vi "Test - LabVIEW-ini Config.vi"() -> ()   [LabVIEW 2021]
uses:
  Sources/Global Config.ctl
  Sources/ini Entry.ctl
  Sources/VIPM.ctl
panel:
  out "text":string
  out "Test Result":bool
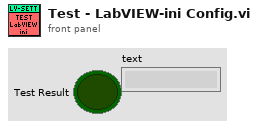
[diagram p1: front panel]
types:
  T1 = enum16{"open", "replace", "create", "open or create", "replace or create", "replace or create with confirmation"}
  T2 = typedef "ini Entry.ctl" = cluster{"section":string, "key":string, "value":variant}
  T3 = typedef "Global Config.ctl" = cluster{"LabVIEW.ini":T2[], "VIPM":T4}
  T4 = typedef "VIPM.ctl" = cluster{"official-packages":string[], "unofficial-package-urls":string[]}
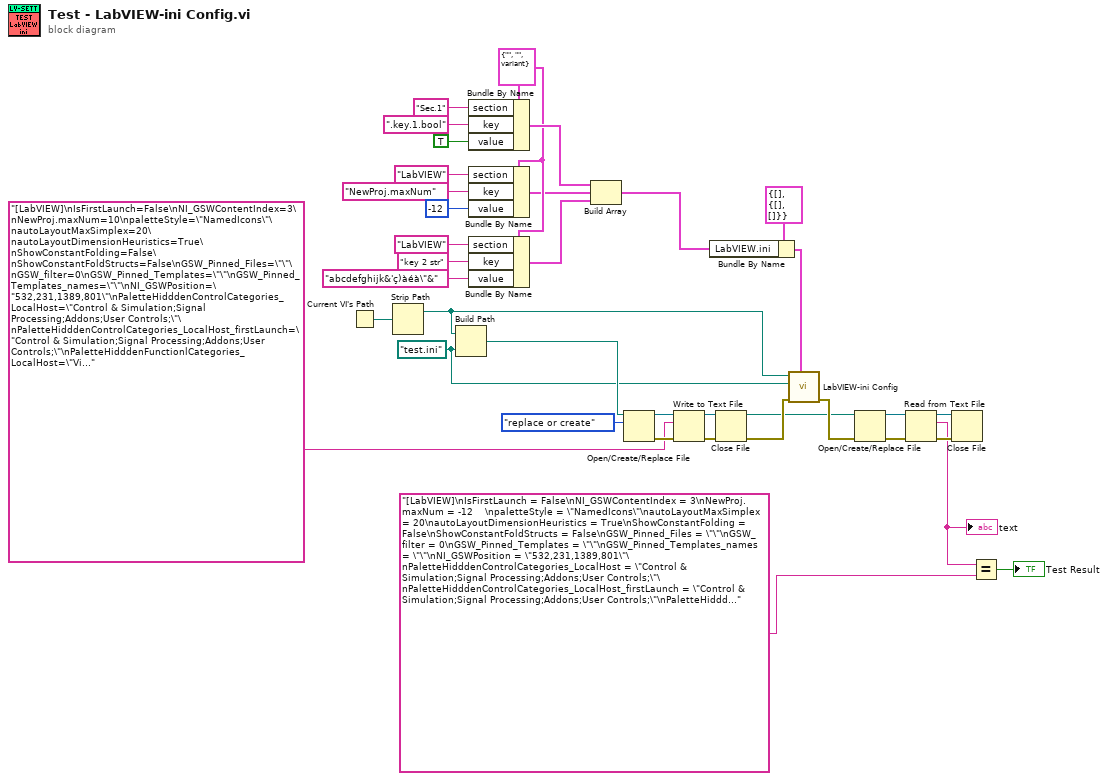
[diagram p0: block diagram]
diagram:
  w12 = path "test.ini" ("name or relative path")
  w24 = T2 {"section"="", "key"="", "value"=variant} ("ini Entry")
  n1 = Current VI's Path() -> (path=w20:path)
  n2 = Strip Path(path=w20) -> (stripped path=w14:path)  [unwired: 1 out]
  n3 = Build Path(base path=w14, name or relative path=w12) -> (appended path=w13:path)
  n4 = Bundle By Name(cluster=w24, "section"="Sec.1", "key"=".key.1.bool", "value"=TRUE) -> (w31:T2)
  n5 = Bundle By Name(cluster=w24, "section"="LabVIEW", "key"="NewProj.maxNum", "value"=-12) -> (w22:T2)
  n6 = Bundle By Name(cluster=w24, "section"="LabVIEW", "key"="key 2 str", "value"="abcdefghijk&'ç)àéà\"&" ("key")) -> (w21:T2)
  n7 = Build Array(w31, w22, w21) -> (w30:T2[])
  n8 = Open/Create/Replace File(file path (use dialog)=w13, operation (0:open)=T1."replace or create") -> (refnum out=w19:refnum<file>, error out=w18:errorcluster)  [unwired: 4 in, 1 out]
  n9 = Write to Text File(file (use dialog)=w19, text="[LabVIEW]\nIsFirstLaunch=False\nNI_GSWContentIndex=3\nNewProj.maxNum=10\npaletteStyle=\"NamedIcons\"\nautoLayoutMaxSimplex=20\nautoLayoutDimensionHeuristics=True\nShowConstantFolding=False\nShowConstantFoldStructs=False\nGSW_Pinned_Files=\"\"\nGSW_filter=0\nGSW_Pinned_Templates=\"\"\nGSW_Pinned_Templates_names=\"\"\nNI_GSWPosition=\"532,231,1389,801\"\nPaletteHidddenControlCategories_LocalHost=\"Control & Simulation;Signal Processing;Addons;User Controls;\"\nPaletteHidddenControlCategories_LocalHost_firstLaunch=\"Control & Simulation;Signal Processing;Addons;User Controls;\"\nPaletteHidddenFunctionlCategories_LocalHost=\"Vision and Motion;Favorites;User Libraries;\"\nPaletteHidddenFunctionlCategories_LocalHost_firstLaunch=\"Vision and Motion;Favorites;User Libraries;\"\nmenuSetup=\"default\"\nsaveFloaterLocations=True\nfind.viListFlags=4\nLastErrorListSize=0,0,0,0\nSaveChanges_ApplyToAll=True\nFancyFPTerms=False\nautoInsertFeedbackNode=False\nDefaultLabelPositionBD=11\nDefaultLabelPositionIndBD=5\nautoLayoutMaxHeuristics=0\nSnapGridDrawAsLines=2\nNISearchCategoryOrder=\"LvHelpSearch;LvPaletteSearch;Web Help;Support;Downloads;Product Information\"\nserver.tcp.enabled=TRUE\nNewProj.RecentLocationPaths=\"C:\\Program Files (x86)\\National Instruments\\LabVIEW 2021\\ProjectTemplates\\Source\\Core\\Blank Project\"\nNewProj.RecentTitles=\"Blank Project\"\nProjectExplorer.ClassicPosition=123,705,523,1076\nNewDlgRecentMainTemplates.pathList=\"\"\nNewDlgSmall=False\nNewDlgCollapsed=\"77E350A8-F9AA-43FF-85E2-454279EBB9A7\t3F7CF7A8-5E4D-4EDC-AA25-FA4A326988EF\t8E4D36AD-F776-4C48-97C6-C1D85EFE889F\"\nNewDlgLastSelected=\"D60740D6-F254-4BBC-5675-8858F35B810E\"\nNewDlgBounds=\"800;600\"\nNewDlgRecentTemplates.pathList=\"\"\nIconEditor.FirstLaunch=False\nIconEditor.TextFont=\"Small Fonts\"\nIconEditor.TextAlignment=00000001\nIconEditor.TextSize=00000009\nIconEditor.Save3rdPartyTemplates=True\nIconEditor.3rdPartyTemplatesFolderName=\"3rd party\"\nIconEditor.TextTab.Color1stBodyLine=00000000\nIconEditor.TextTab.Color2ndBodyLine=00000000\nIconEditor.TextTab.Color3tdBodyLine=00000000\nIconEditor.TextTab.Color4thBodyLine=00000000\nIconEditor.TextTab.TextFont=\"Small Fonts\"\nIconEditor.TextTab.TextAlignment=00000001\nIconEditor.TextTab.TextSize=00000009\nIconEditor.TextTab.Options=00000001\nIconEditor.FillColor=00F6F6F6\nIconEditor.EdgeColor=00FF7F7F\nIconEditor.Tool=00000003\nIconEditor.ShowLayerTab=True\nIconEditor.ShowTerminals=False\nIconEditor.SaveLayersWithVI=False\nIconEditor.MostRecentTab=00000001\nIconEditor.Position=\"472,281,1448,752\"\nContextHelpLoc=17,1639,197,1910\ncolorHistoryItemA=00FFFFFF\ncolorHistoryItemB=0000FF80\nserver.tcp.port=3363\nserver.tcp.access=\"+127.0.0.1;+localhost;+*\"\nmenuKeywordExtra=412\nQuickDropPosition=\"795,392,1125,640\"\nsimpleDiagramHelp=False\nNoAdvice070=\",CleanUpWire\"\n", error in=w18) -> (refnum out=w17:refnum<file>, error out=w16:errorcluster)  [unwired: 1 in, 1 out]
  n10 = Bundle By Name(cluster=T3 {"LabVIEW.ini"=[], "VIPM"={"official-packages"=[], "unofficial-package-urls"=[]}} ("Global Config"), "LabVIEW.ini"=w30) -> (w35:T3)
  n11 = Close File(refnum=w17, error in=w16) -> (path=w8:path, error out=w11:errorcluster)
  n12 = call "LabVIEW-ini Config.vi"("Global Config"=w35, "error in"=w11, "ini Name (LabVIEW.ini)"=w12, "LabVIEW Install Folder"=w14) -> ("error out"=w9:errorcluster)  [unwired: 7 in]
  n13 = Open/Create/Replace File(file path (use dialog)=w8, error in=w9) -> (refnum out=w7:refnum<file>, error out=w6:errorcluster)  [unwired: 4 in, 1 out]
  n14 = Read from Text File(file (use dialog)=w7, error in=w6) -> (refnum out=w5:refnum<file>, text=w3:string, error out=w4:errorcluster)  [unwired: 2 in, 1 out]
  "text" <- w3
  n15 = Close File(refnum=w5, error in=w4) -> ()  [unwired: 2 out]
  n16 = Equal?(x=w3, y="[LabVIEW]\nIsFirstLaunch = False\nNI_GSWContentIndex = 3\nNewProj.maxNum = -12    \npaletteStyle = \"NamedIcons\"\nautoLayoutMaxSimplex = 20\nautoLayoutDimensionHeuristics = True\nShowConstantFolding = False\nShowConstantFoldStructs = False\nGSW_Pinned_Files = \"\"\nGSW_filter = 0\nGSW_Pinned_Templates = \"\"\nGSW_Pinned_Templates_names = \"\"\nNI_GSWPosition = \"532,231,1389,801\"\nPaletteHidddenControlCategories_LocalHost = \"Control & Simulation;Signal Processing;Addons;User Controls;\"\nPaletteHidddenControlCategories_LocalHost_firstLaunch = \"Control & Simulation;Signal Processing;Addons;User Controls;\"\nPaletteHidddenFunctionlCategories_LocalHost = \"Vision and Motion;Favorites;User Libraries;\"\nPaletteHidddenFunctionlCategories_LocalHost_firstLaunch = \"Vision and Motion;Favorites;User Libraries;\"\nmenuSetup = \"default\"\nsaveFloaterLocations = True\nfind.viListFlags = 4\nLastErrorListSize = 0,0,0,0\nSaveChanges_ApplyToAll = True\nFancyFPTerms = False\nautoInsertFeedbackNode = False\nDefaultLabelPositionBD = 11\nDefaultLabelPositionIndBD = 5\nautoLayoutMaxHeuristics = 0\nSnapGridDrawAsLines = 2\nNISearchCategoryOrder = \"LvHelpSearch;LvPaletteSearch;Web Help;Support;Downloads;Product Information\"\nserver.tcp.enabled = TRUE\nNewProj.RecentLocationPaths = \"C:\\Program Files (x86)\\National Instruments\\LabVIEW 2021\\ProjectTemplates\\Source\\Core\\Blank Project\"\nNewProj.RecentTitles = \"Blank Project\"\nProjectExplorer.ClassicPosition = 123,705,523,1076\nNewDlgRecentMainTemplates.pathList = \"\"\nNewDlgSmall = False\nNewDlgCollapsed = \"77E350A8-F9AA-43FF-85E2-454279EBB9A7\t3F7CF7A8-5E4D-4EDC-AA25-FA4A326988EF\t8E4D36AD-F776-4C48-97C6-C1D85EFE889F\"\nNewDlgLastSelected = \"D60740D6-F254-4BBC-5675-8858F35B810E\"\nNewDlgBounds = \"800;600\"\nNewDlgRecentTemplates.pathList = \"\"\nIconEditor.FirstLaunch = False\nIconEditor.TextFont = \"Small Fonts\"\nIconEditor.TextAlignment = 00000001\nIconEditor.TextSize = 00000009\nIconEditor.Save3rdPartyTemplates = True\nIconEditor.3rdPartyTemplatesFolderName = \"3rd party\"\nIconEditor.TextTab.Color1stBodyLine = 00000000\nIconEditor.TextTab.Color2ndBodyLine = 00000000\nIconEditor.TextTab.Color3tdBodyLine = 00000000\nIconEditor.TextTab.Color4thBodyLine = 00000000\nIconEditor.TextTab.TextFont = \"Small Fonts\"\nIconEditor.TextTab.TextAlignment = 00000001\nIconEditor.TextTab.TextSize = 00000009\nIconEditor.TextTab.Options = 00000001\nIconEditor.FillColor = 00F6F6F6\nIconEditor.EdgeColor = 00FF7F7F\nIconEditor.Tool = 00000003\nIconEditor.ShowLayerTab = True\nIconEditor.ShowTerminals = False\nIconEditor.SaveLayersWithVI = False\nIconEditor.MostRecentTab = 00000001\nIconEditor.Position = \"472,281,1448,752\"\nContextHelpLoc = 17,1639,197,1910\ncolorHistoryItemA = 00FFFFFF\ncolorHistoryItemB = 0000FF80\nserver.tcp.port = 3363\nserver.tcp.access = \"+127.0.0.1;+localhost;+*\"\nmenuKeywordExtra = 412\nQuickDropPosition = \"795,392,1125,640\"\nsimpleDiagramHelp = False\nNoAdvice070 = \",CleanUpWire\"\nkey 2 str = \"abcdefghijk&'ç)àéà\"&\"\n\n[Sec.1]\n.key.1.bool = TRUE" ("text")) -> (x = y?=→"Test Result":bool)
